vi "Kalman CalculationVelCmd.vi"(0 "Lado":enum16{"Esquerdo", "Direito"}(ring) caption="Enum", 4 "our_robots":bool=TRUE, 5 "u_k":T1, 6 "R":T1=[[0.1, 0.0, 0.0], [0.0, 0.1, 0.0], [0.0, 0.0, 0.1]], 7 "Use Observation":bool=TRUE, 8 "intervalo":dbl=1.0, 9 "Pk-1|k-1":T1, 10 "x_k-1|k-1":T1=[[0.0, 0.0, 0.0], [0.0, 0.0, 0.0], [0.0, 0.0, 0.0]], 11 "z_k":T1) -> (1 "Conf":dbl, 2 "Pk|k":T1, 3 "x_k|k":T1)   [LabVIEW 2018]
uses:
  <vilib>/Analysis/Matrix/Datatypes/RealMatrix.ctl
  <vilib>/Analysis/_algsub.llb/Real Matrix Norm.vi
  <vilib>/Analysis/Matrix/Numeric/Multiply/Multiply - RM,R.vi
  <vilib>/Analysis/Matrix/Numeric/Conversions/Array To Matrix - RA2.vi
  <vilib>/Analysis/Matrix/Numeric/Multiply/Multiply - RM,RM.vi
  <vilib>/Analysis/Matrix/Numeric/Add/Add - RM,RM.vi
  <vilib>/Analysis/Matrix/NI_Matrix.lvlib
  <vilib>/Analysis/NI_AALBase.lvlib
  <vilib>/Analysis/baseanly.llb/Real Inverse Matrix.vi
  <vilib>/Analysis/NI_AALPro.lvlib
panel:
  out "In Range?":bool[][](array[boolean])
  in  "DesAccel_Max":dbl=5.0
  in  "zero":T1=[[0.0], [0.0], [0.0], [0.0], [0.0], [0.0]]
  in  "Accel_Max":dbl=5.0 format="%#_13g"
  out "appended array":T1
  out "K_k":T1
  out "Inverse Matrix":T1
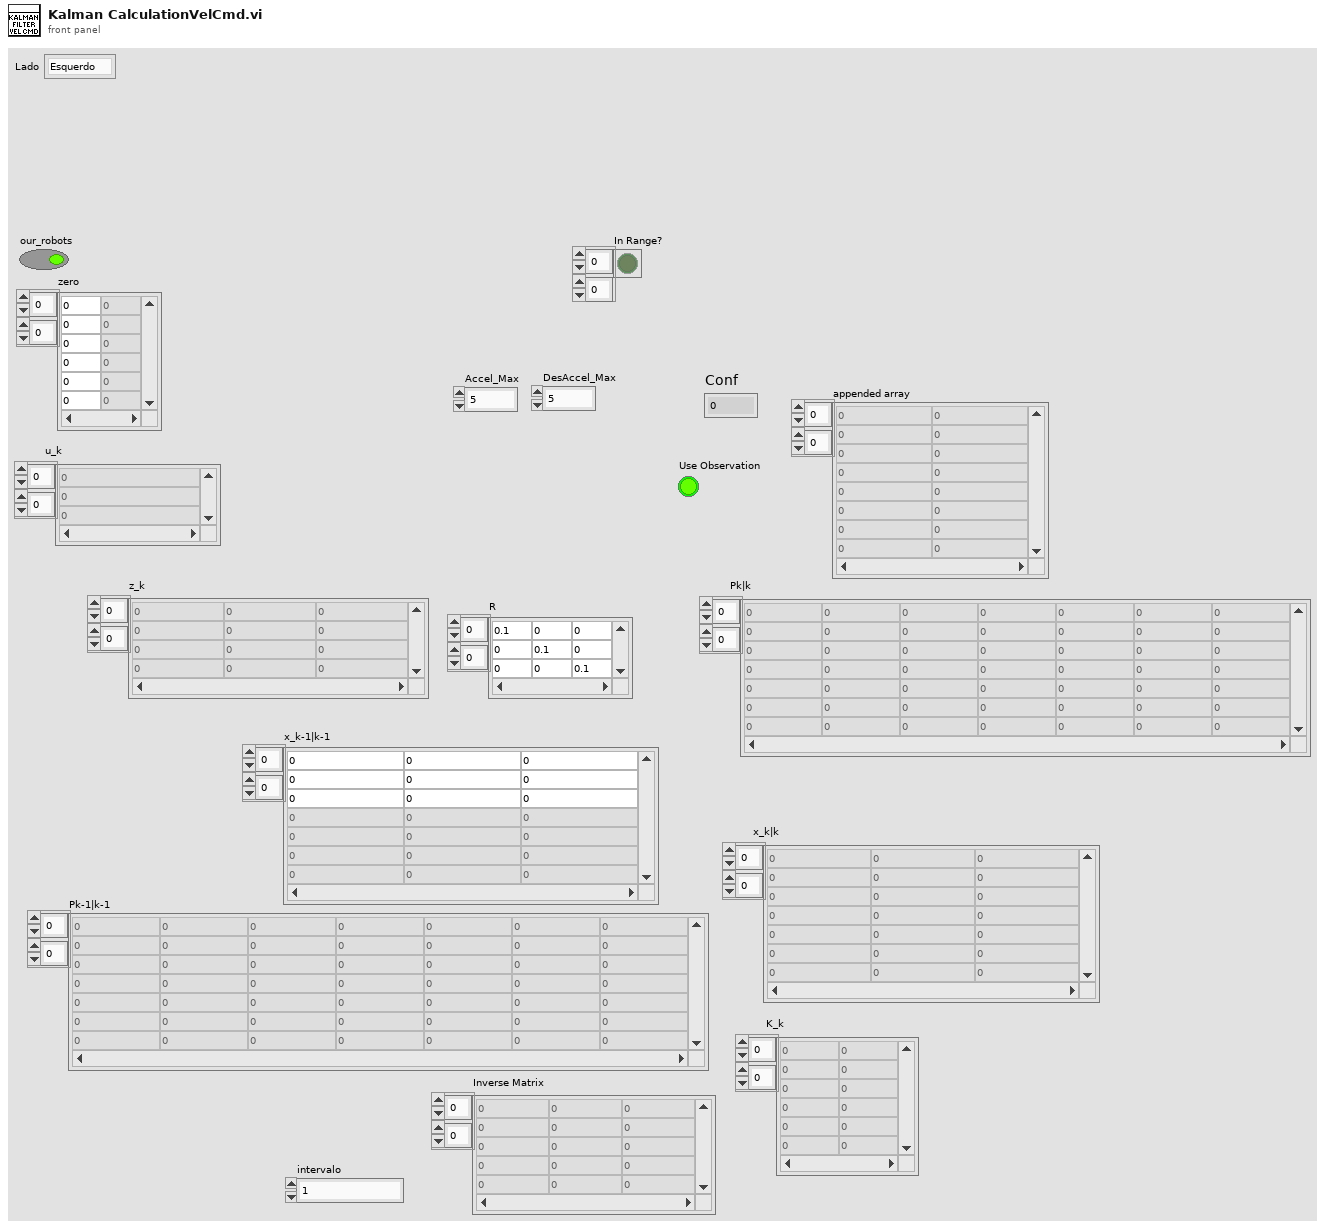
[diagram p1: front panel]
types:
  T1 = typedef "NI_Matrix.lvlib/RealMatrix.ctl" = dbl[][]
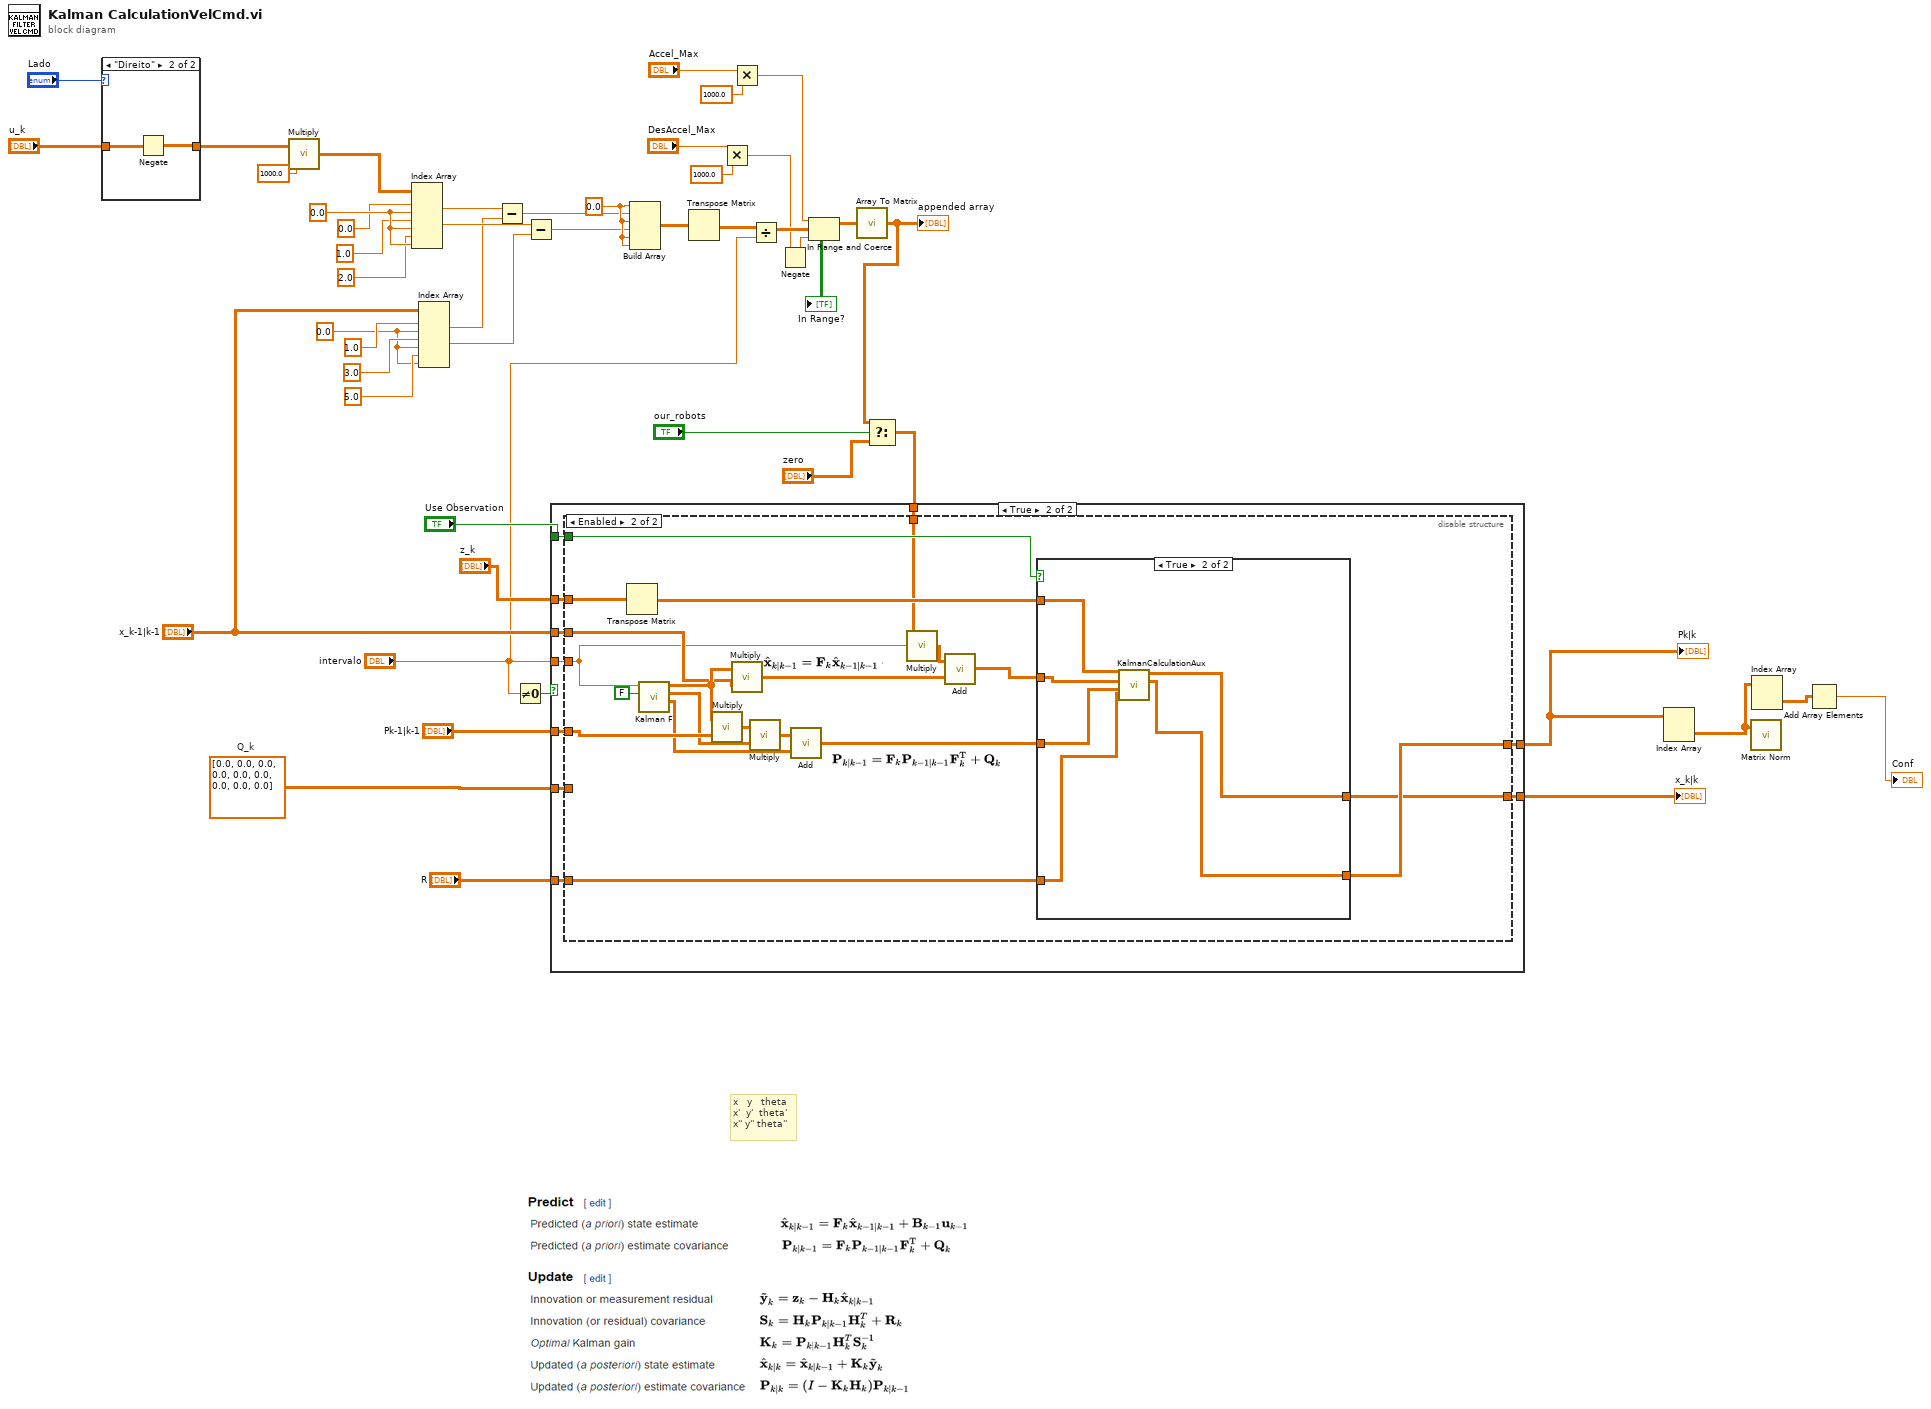
[diagram p0: block diagram]
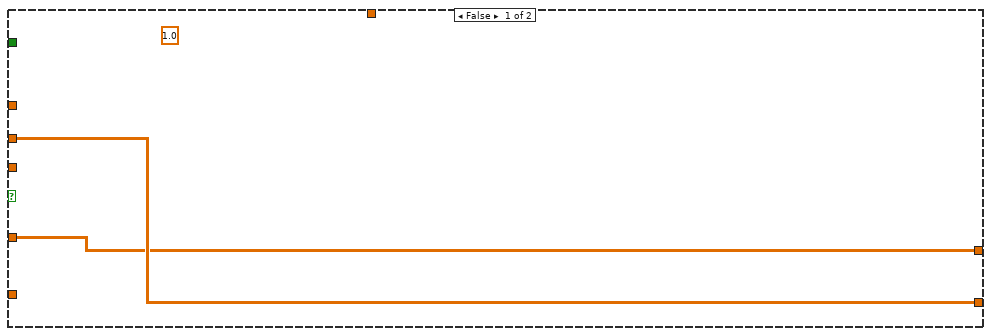
[diagram p3: hidden frame]
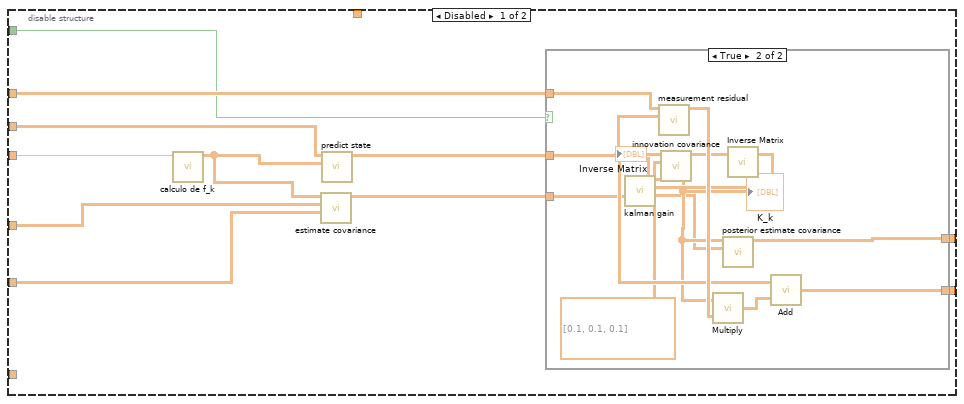
[diagram p4: hidden frame]
diagram:
  w29 = 0.0
  w37 = 0.0
  w38 = 0.0
  w46 = T1 [[0.0, 0.0, 0.0], [0.0, 0.0, 0.0], [0.0, 0.0, 0.0]]  # Q_k
  # "x   y   theta\nx'  y'  theta'\nx'' y'' theta''"
  n1 = case shown="\"Direito\"" "Lado" {
    tunnel: [w50 w51] -> w2
    tunnel: "u_k" -> [w50 w52]
    frame "Esquerdo", Default {
    }
    frame "Direito" {
      n2 = Negate(x=w52) -> (-x=w51:T1)
    }
  }
  n3 = call-poly <vilib>:"Multiply.vi"("Real Scalar c"=1000.0, "Real Matrix A"=w2) -> ("A * c"=w11:T1)
  n4 = Index Array(array=w11, index (row) #1=0.0, index (col) #1=w38, index (row) #2=1.0, index (col) #2=w38, index (row) #3=2.0, index (col) #3=w38) -> (element #1=w24:dbl, element #2=w27:dbl)  [unwired: 1 out]
  n5 = Index Array(array="x_k-1|k-1", index (row) #1=1.0, index (col) #1=w29, index (row) #2=3.0, index (col) #2=w29, index (row) #3=5.0, index (col) #3=w29) -> (element #1=w25:dbl, element #2=w26:dbl)  [unwired: 1 out]
  n6 = Subtract(x=w24, y=w25) -> (x-y=w23:dbl)
  n7 = Not Equal To 0?(x="intervalo") -> (x != 0?=w47:bool)
  n8 = Subtract(x=w27, y=w26) -> (x-y=w22:dbl)
  n9 = Build Array(w37, w23, w37, w22, w37, w37) -> (w33:T1)
  n10 = Transpose Matrix(1:w33) -> (0:w21:T1)
  n11 = Multiply ("Multiply.vi")(x="DesAccel_Max", y=1000.0) -> (x*y=w4:dbl)
  n12 = Multiply ("Multiply.vi")(x="Accel_Max", y=1000.0) -> (x*y=w7:dbl)
  n13 = Divide(x=w21, y="intervalo") -> (x/y=w20:T1)
  n14 = Negate(x=w4) -> (-x=w13:dbl)
  n15 = In Range and Coerce(upper limit=w7, x=w20, lower limit=w13) -> (coerced(x)=w19:dbl[][], In Range?=→"In Range?":bool[][])
  n16 = call-poly <vilib>:"Array To Matrix.vi"("Real 2D Array"=w19) -> ("Real Matrix"=w17:T1)
  "appended array" <- w17
  n17 = Select(t=w17, s="our_robots", f="zero") -> (s? t:f=w15:T1)
  n18 = case shown="True" w47 {
    tunnel: "intervalo" -> [_ w64]
    tunnel: [w54 w63] -> w39
    tunnel: "Pk-1|k-1" -> [w53 w62]
    tunnel: "x_k-1|k-1" -> [w54 w60]
    tunnel: [w53 w61] -> w48
    tunnel: w46 -> [_ w59]
    tunnel: "z_k" -> [_ w58]
    tunnel: "Use Observation" -> [_ w57]
    tunnel: "R" -> [_ w56]
    tunnel: w15 -> [_ w55]
    frame False {
      (unwired) 1.0 ("intervalo")
    }
    frame True {
      n19 = disable-structure shown="Enabled" {
        disable-tunnel: w64 -> [w75 w91]
        disable-tunnel: [w72 w99] -> w63
        disable-tunnel: w62 -> [w71 w108]
        disable-tunnel: [w70 w100] -> w61
        disable-tunnel: w60 -> [w69 w97]
        disable-tunnel: w59 -> [w67 _]
        disable-tunnel: w58 -> [w66 w103]
        disable-tunnel: w57 -> [w65 w95]
        disable-tunnel: w56 -> [_ w96]
        disable-tunnel: w55 -> [_ w92]
        frame Disabled {
          n20 = call "calculo de f_k.vi"("iteração"=w75) -> ("F_k"=w68:T1)  [unwired: 10 in]
          n21 = call "estimate covariance.vi"("Q_k"=w67, "Pk-1|k-1"=w71, "F_k"=w68) -> ("Pk|k-1"=w73:T1)  [unwired: 8 in]
          n22 = call "predict state.vi"("F_k"=w68, "x_k-1|k-1"=w69) -> ("x_k|k-1"=w74:T1)  [unwired: 9 in]
          n23 = case shown="True" w65 {
            tunnel: [w77 w87] -> w72
            tunnel: w74 -> [w77 w85]
            tunnel: [w76 w82] -> w70
            tunnel: w73 -> [w76 w80]
            tunnel: w66 -> [_ w79]
            frame False {
            }
            frame True {
              n24 = call "measurement residual.vi"("x_k|k-1"=w85, "z_k"=w79) -> ("y~_k"=w86:T1)  [unwired: 9 in]
              n25 = call "innovation covariance.vi"("R"=T1 [[0.1, 0.1, 0.1]], "Pk|k-1"=w80) -> ("S_k"=w84:T1)  [unwired: 8 in, 1 out]
              n26 = call-poly <vilib>:"Inverse Matrix.vi"("Input Matrix"=w84) -> ("Inverse Matrix"=w83:T1)  [unwired: 1 in, 1 out]
              "Inverse Matrix" <- w83
              n27 = call "kalman gain.vi"("Pk|k-1"=w80, "S^-1"=w83) -> ("K_k"=w81:T1)  [unwired: 9 in]
              "K_k" <- w81
              n28 = call-poly <vilib>:"Multiply.vi"("Real Matrix B"=w86, "Real Matrix A"=w81) -> ("A * B"=w88:T1)
              n29 = call "posterior estimate covariance.vi"("Pk|k-1"=w80, "K_k"=w81) -> ("Pk|k"=w82:T1)  [unwired: 9 in]
              n30 = call-poly <vilib>:"Add.vi"("Real Matrix B"=w88, "Real Matrix A"=w85) -> ("A + B"=w87:T1)
            }
          }
        }
        frame Enabled {
          n31 = Transpose Matrix(1:w103) -> (0:w102:T1)
          n32 = call "Kalman F.vi"("Ball?"=FALSE, "intervalo"=w91) -> ("Q"=w104:T1, "F'"=w106:T1, "F"=w98:T1)  [unwired: 7 in]
          n33 = call-poly <vilib>:"Multiply.vi"("Real Matrix B"=w108, "Real Matrix A"=w98) -> ("A * B"=w107:T1)
          n34 = call-poly <vilib>:"Multiply.vi"("Real Matrix B"=w97, "Real Matrix A"=w98) -> ("A * B"=w90:T1)
          n35 = call-poly <vilib>:"Multiply.vi"("Real Matrix B"=w106, "Real Matrix A"=w107) -> ("A * B"=w105:T1)
          n36 = call-poly <vilib>:"Add.vi"("Real Matrix B"=w104, "Real Matrix A"=w105) -> ("A + B"=w101:T1)
          n37 = call-poly <vilib>:"Multiply.vi"("Real Scalar c"=w91, "Real Matrix A"=w92) -> ("A * c"=w93:T1)
          n38 = call-poly <vilib>:"Add.vi"("Real Matrix B"=w90, "Real Matrix A"=w93) -> ("A + B"=w94:T1)
          n39 = case shown="True" w95 {
            tunnel: w102 -> [_ w116]
            tunnel: w94 -> [w110 w111]
            tunnel: w101 -> [w109 w115]
            tunnel: [w109 w112] -> w100
            tunnel: [w110 w113] -> w99
            tunnel: w96 -> [_ w114]
            frame False {
            }
            frame True {
              n40 = call "KalmanCalculationAux.vi"("R"=w114, "A + B in"=w115, "A + B 3"=w111, "z_k"=w116) -> ("A - B"=w112:T1, "A + B out"=w113:T1)  [unwired: 6 in]
            }
          }
        }
      }
    }
  }
  "Pk|k" <- w48
  "x_k|k" <- w39
  n41 = Index Array(array=w48) -> (element=w42:T1)  [unwired: 2 in]
  n42 = call-poly <vilib>:"Matrix Norm.vi"("Input Matrix"=w42) -> ()  [unwired: 1 in, 2 out]
  n43 = Index Array(array=w42) -> (element=w41:T1)  [unwired: 2 in]
  n44 = Add Array Elements(numeric array=w41) -> (sum=→"Conf":dbl)
